vi "EXCOM-TCP-WRITE.vi"(5 "Args":dbl[](array[numeric]) format="%.2f", 6 "Commande #":i32=-1, 7 "Error IN":errorcluster, 10 "connection ID":refnum<k5>) -> (0 "Error OUT":errorcluster, 1 "OK Done":bool, 2 "Cmd String":string, 3 "connection ID out":refnum<k5>)   [LabVIEW 2011]
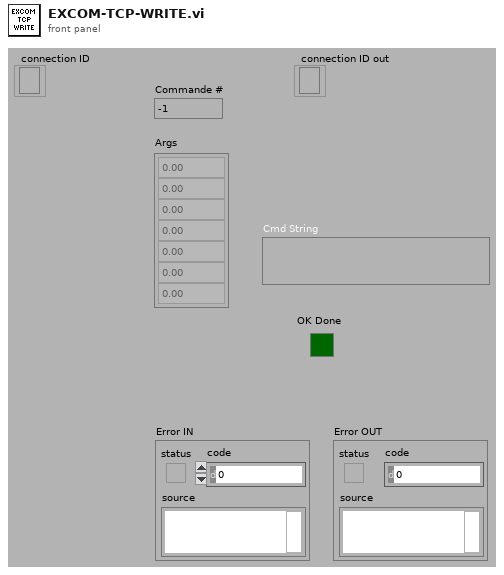
[diagram p1: front panel]
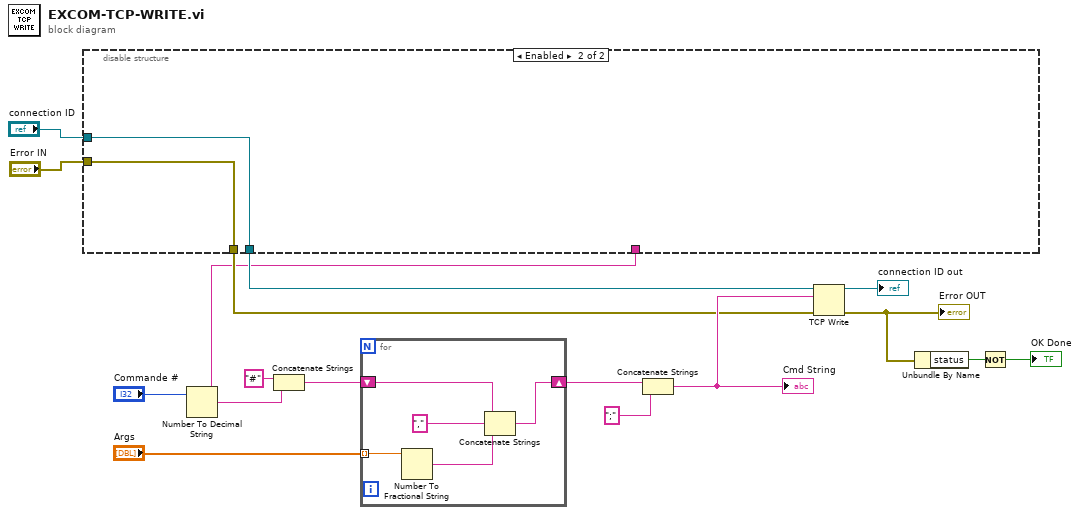
[diagram p0: block diagram]
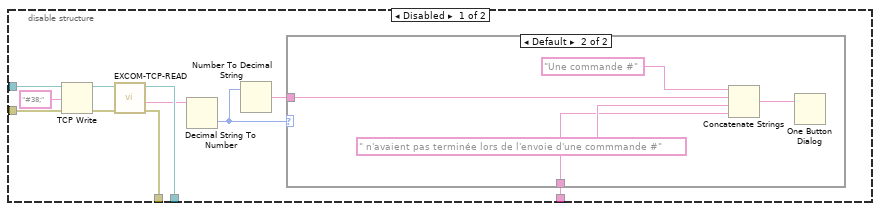
[diagram p2: hidden frame]
diagram:
  n1 = Number To Decimal String(number="Commande #") -> (decimal integer string=w1:string)  [unwired: 1 in]
  n2 = disable-structure shown="Enabled" {
    disable-tunnel: "connection ID" -> [w27 w34]
    disable-tunnel: "Error IN" -> [w26 w33]
    disable-tunnel: [w23 w34] -> w3
    disable-tunnel: [w22 w33] -> w2
    disable-tunnel: w1 -> [w20 _]
    frame Disabled {
      n3 = TCP Write(connection ID=w27, data in="#38;", error in (no error)=w26) -> (connection ID out=w25:refnum<k5>, error out=w24:errorcluster)  [unwired: 1 in, 1 out]
      n4 = call "EXCOM-TCP-READ.vi"("Error In"=w24, "connection ID"=w25) -> ("Error Out"=w22:errorcluster, "Response"=w19:string, "CID Out"=w23:refnum<k5>)  [unwired: 5 in]
      n5 = Decimal String To Number(string=w19) -> (number=w18:i32)  [unwired: 2 in, 1 out]
      n6 = Number To Decimal String(number=w18) -> (decimal integer string=w17:string)  [unwired: 1 in]
      n7 = case shown="Default" w18 {
        tunnel: w20 -> [_ w30]
        tunnel: w17 -> [_ w29]
        frame 0 {
        }
        frame Default {
          n8 = Concatenate Strings("Une commande #", w29, " n'avaient pas terminée lors de l'envoie d'une commmande #" ("string"), w30) -> (w28:string)
          n9 = One Button Dialog(message=w28) -> ()  [unwired: 1 in, 1 out]
        }
      }
    }
    frame Enabled {
    }
  }
  n10 = Concatenate Strings("#" ("string"), w1) -> (w13:string)
  n11 = for {
    shift-right: [w39] -> w8
    shift-left: w13 -> [w37]
    tunnel: "Args" -> [w38] mode=indexing
    n12 = Number To Fractional String(number=w38) -> (F-format string=w35:string)  [unwired: 3 in]
    n13 = Concatenate Strings(w37, ",", w35) -> (w39:string)
  }
  n14 = Concatenate Strings(w8, ";" ("string")) -> (w6:string)
  "Cmd String" <- w6
  n15 = TCP Write(connection ID=w3, data in=w6, error in (no error)=w2) -> (connection ID out=→"connection ID out":refnum<k5>, error out=w11:errorcluster)  [unwired: 1 in, 1 out]
  "Error OUT" <- w11
  n16 = Unbundle By Name(w11) -> ("status"=w10:bool)
  n17 = Not(x=w10) -> (.not. x?=→"OK Done":bool)
